vi "Know Position.vi"(0 "Ref_Drive 1R":T1, 1 "Ref_Drive 2R":T1, 2 "Ref_Drive 3R":T1, 3 "Ref_Drive 4L":T1, 4 "Ref_Drive 5L":T1, 5 "Ref_Drive 6L":T1) -> ()   [LabVIEW 2018]
uses:
  <vilib>/Rock Robotics/WPI/MotorControl/WPI_MotorControlDeviceRef.ctl
  <vilib>/Rock Robotics/WPI/MotorControl/WPI_MotorControlType.ctl
  <vilib>/Rock Robotics/SystemInterfaces/DIO/FPGA_DIOPWMChannel.ctl
  <vilib>/Rock Robotics/WPI/PWM/WPI_PWMDeadband.ctl
  <vilib>/Rock Robotics/SystemInterfaces/DIO/FPGA_DIOChannel.ctl
  Robot States.vi
  Sensor Readings.vi
panel:
  out "XY Graph":cluster{dbl[], dbl[]}(graph)
  in  "Reset Positon":bool
  out "Heading (deg)":dbl format="%#_13g"
  out "Y Position (in)":dbl
  out "X Position (in)":dbl
  in  "Plot Drive Encoder Data":bool
  out "Drive Encoder Velocities":cluster{dbl, dbl}
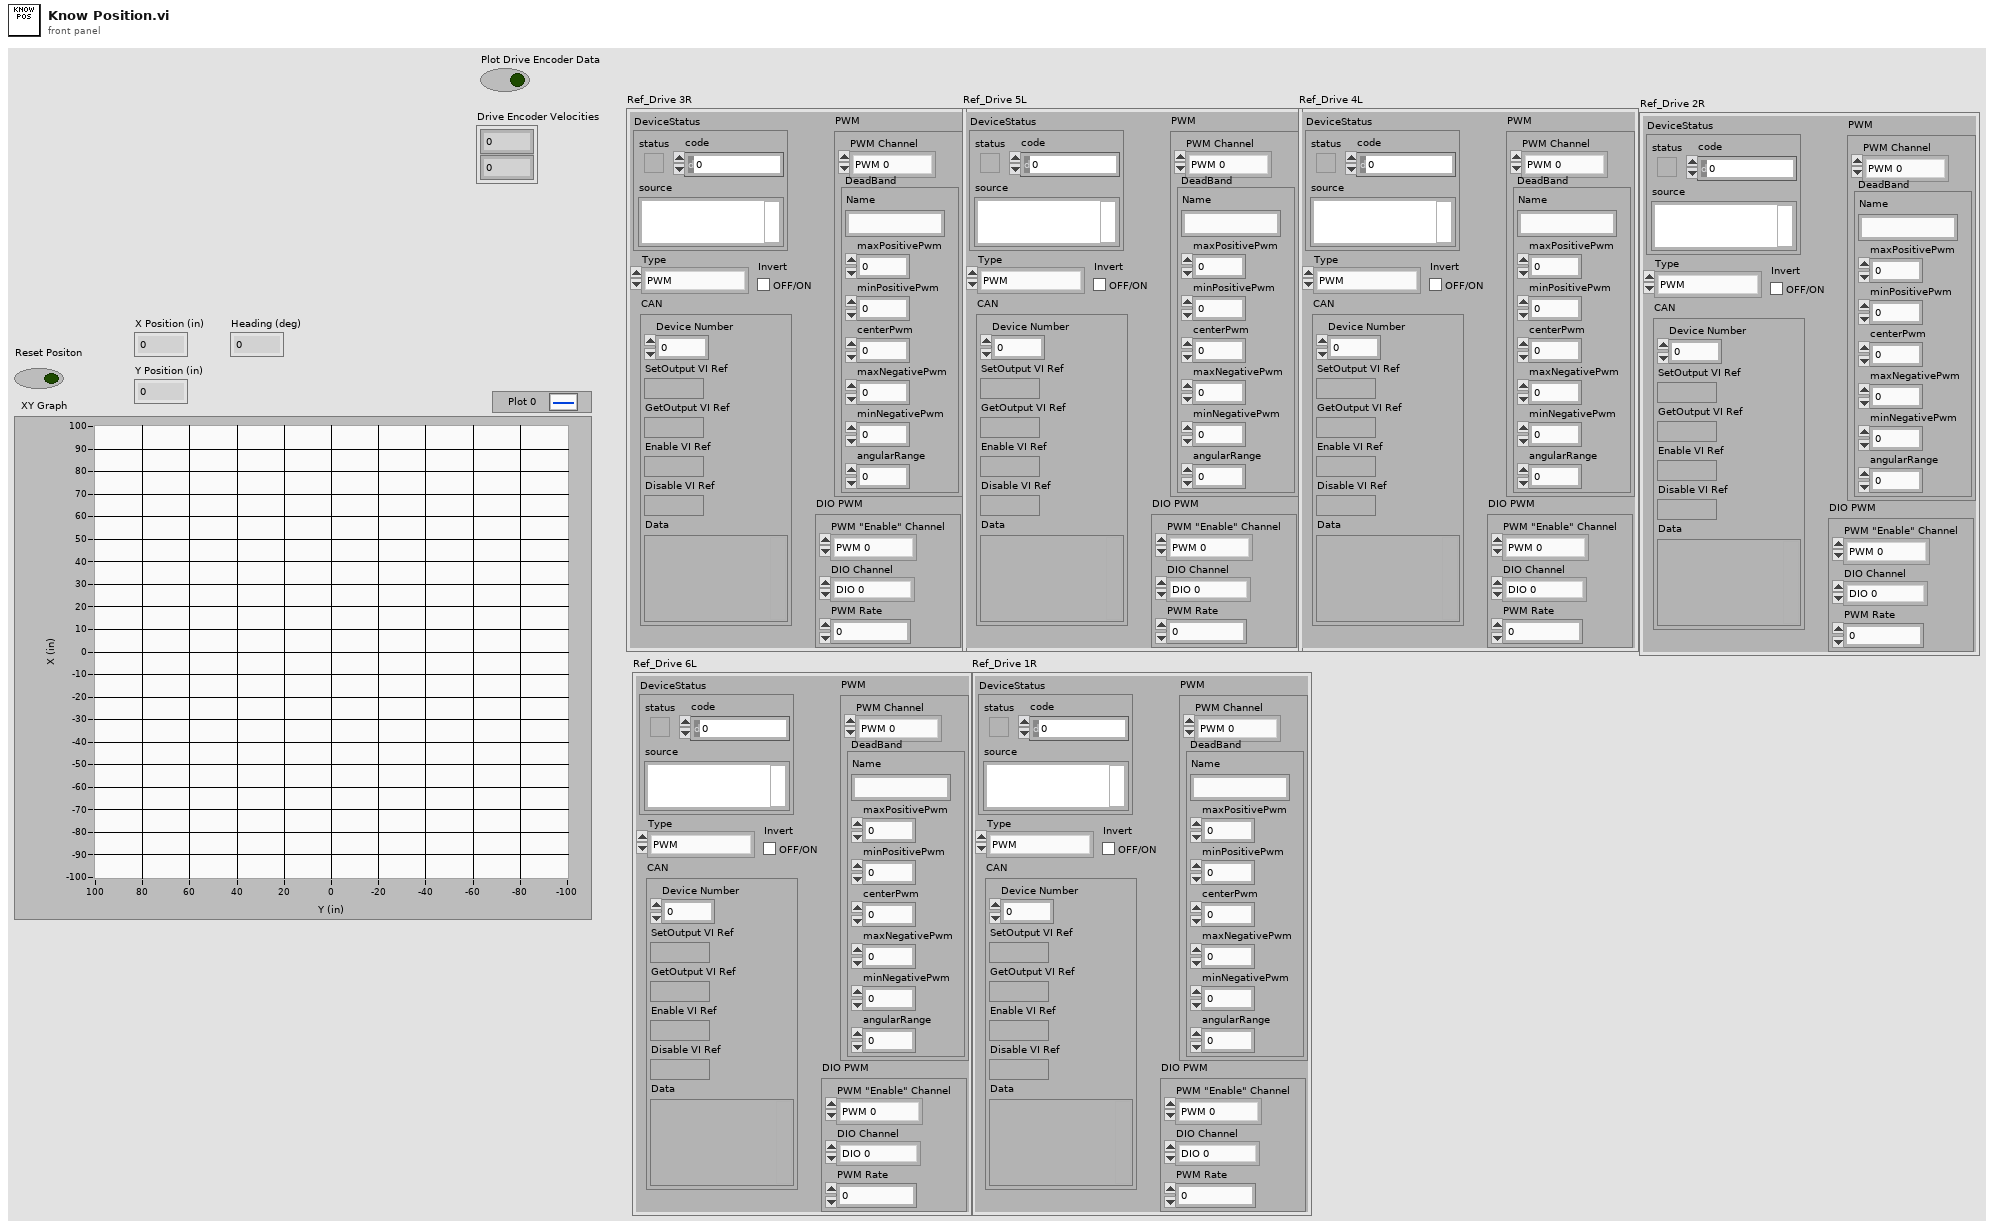
[diagram p1: front panel]
types:
  T1 = typedef "WPI_MotorControlDeviceRef.ctl" = cluster{"DeviceStatus":errorcluster, "Type":T2, "PWM":cluster{"PWM Channel":T3, "DeadBand":T4}, "CAN":cluster{"Device Number":u8, "SetOutput VI Ref":variant, "GetOutput VI Ref":variant, "Enable VI Ref":variant, "Disable VI Ref":variant, "Data":variant}, "Invert":bool, "DIO PWM":cluster{"PWM \"Enable\" Channel":T3, "DIOChannel":T5, "PWM Rate":dbl}}
  T2 = typedef "WPI_MotorControlType.ctl" = enum16{"PWM", "CAN", "DIO PWM"}
  T3 = typedef "FPGA_DIOPWMChannel.ctl" = enum8{"PWM 0", "PWM 1", "PWM 2", "PWM 3", "PWM 4", "PWM 5", "PWM 6", "PWM 7", "PWM 8", "PWM 9", "PWM MXP 0", "PWM MXP 1", "PWM MXP 2", "PWM MXP 3", "PWM MXP 4", "PWM MXP 5", "PWM MXP 6", "PWM MXP 7", "PWM MXP 8", "PWM MXP 9", "Invalid"}
  T4 = typedef "WPI_PWMDeadband.ctl" = cluster{"Name":string, "maxPositivePwm":i32, "minPositivePwm":i32, "centerPwm":i32, "maxNegativePwm":i32, "minNegativePwm":i32, "angularRange":u16}
  T5 = typedef "FPGA_DIOChannel.ctl" = enum8{"DIO 0", "DIO 1", "DIO 2", "DIO 3", "DIO 4", "DIO 5", "DIO 6", "DIO 7", "DIO 8", "DIO 9", "DIO MXP 0", "DIO MXP 1", "DIO MXP 2", "DIO MXP 3", "DIO MXP 4", "DIO MXP 5", "DIO MXP 6", "DIO MXP 7", "DIO MXP 8", "DIO MXP 9", "DIO MXP 10", "DIO MXP 11", "DIO MXP 12", "DIO MXP 13", "DIO MXP 14", "DIO MXP 15", "SPI Port CS1", "SPI Port CS2", "SPI Port CS3", "SPI Port MISO", "SPI Port MOSI", "Invalid"}
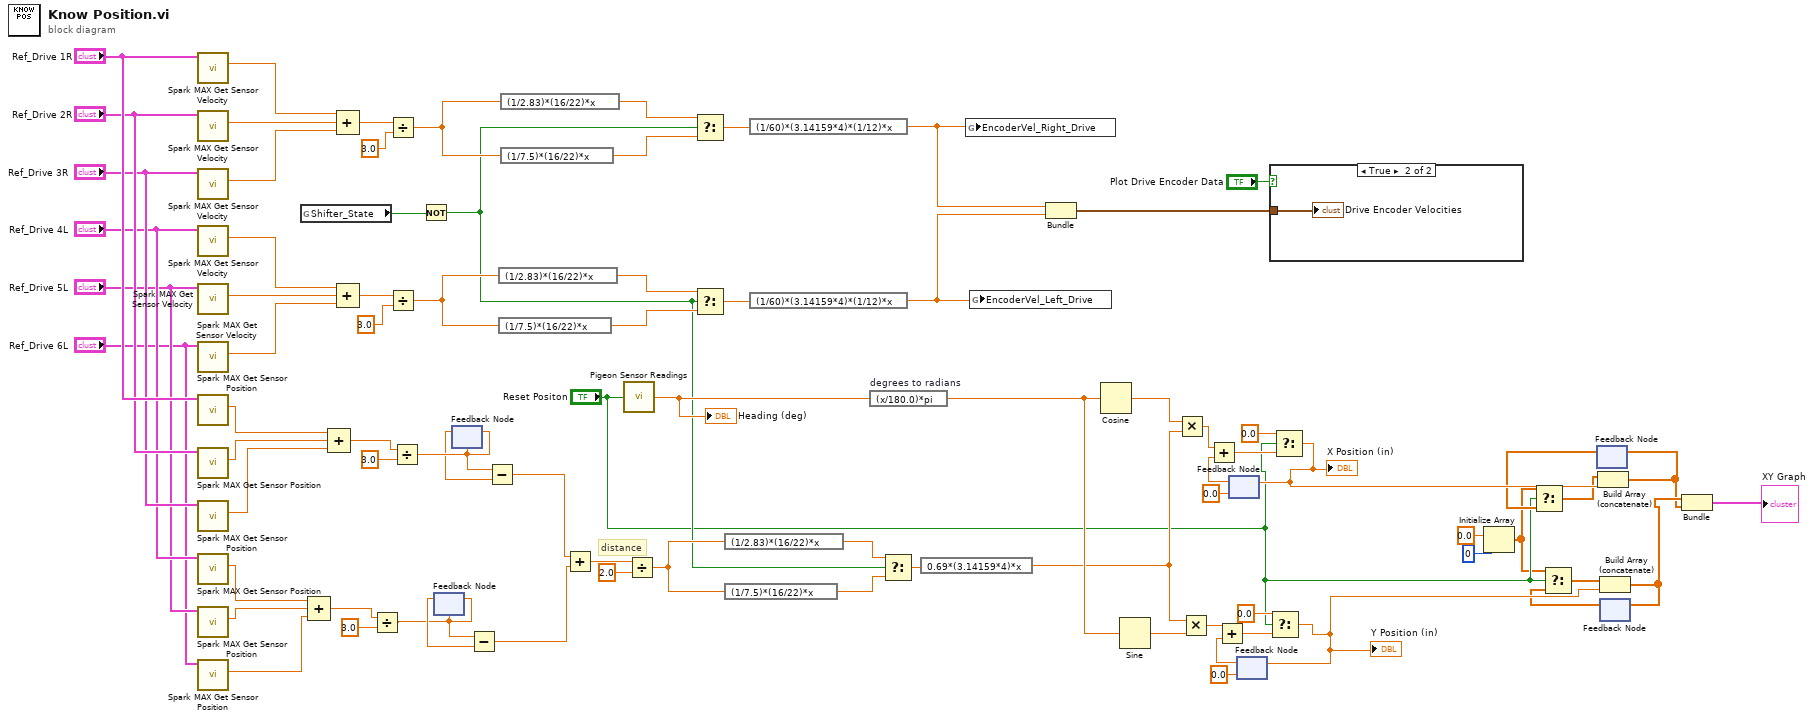
[diagram p0: block diagram]
diagram:
  # "distance"
  n1 = call <vilib>:"Spark MAX Get Sensor Velocity.vi"("MotorControlDevRef in"="Ref_Drive 1R") -> ("Sensor Velocity"=w80:dbl)  [unwired: 7 in, 3 out]
  n2 = call <vilib>:"Spark MAX Get Sensor Velocity.vi"("MotorControlDevRef in"="Ref_Drive 2R") -> ("Sensor Velocity"=w79:dbl)  [unwired: 7 in, 3 out]
  n3 = call <vilib>:"Spark MAX Get Sensor Velocity.vi"("MotorControlDevRef in"="Ref_Drive 3R") -> ("Sensor Velocity"=w78:dbl)  [unwired: 7 in, 3 out]
  n4 = call <vilib>:"Spark MAX Get Sensor Velocity.vi"("MotorControlDevRef in"="Ref_Drive 4L") -> ("Sensor Velocity"=w77:dbl)  [unwired: 7 in, 3 out]
  n5 = call <vilib>:"Spark MAX Get Sensor Velocity.vi"("MotorControlDevRef in"="Ref_Drive 5L") -> ("Sensor Velocity"=w76:dbl)  [unwired: 7 in, 3 out]
  n6 = call <vilib>:"Spark MAX Get Sensor Velocity.vi"("MotorControlDevRef in"="Ref_Drive 6L") -> ("Sensor Velocity"=w75:dbl)  [unwired: 7 in, 3 out]
  n7 = call <vilib>:"Spark MAX Get Sensor Position.vi"("MotorControlDevRef in"="Ref_Drive 1R") -> ("Sensor Position"=w51:dbl)  [unwired: 7 in, 3 out]
  n8 = call <vilib>:"Spark MAX Get Sensor Position.vi"("MotorControlDevRef in"="Ref_Drive 2R") -> ("Sensor Position"=w50:dbl)  [unwired: 7 in, 3 out]
  n9 = call <vilib>:"Spark MAX Get Sensor Position.vi"("MotorControlDevRef in"="Ref_Drive 3R") -> ("Sensor Position"=w49:dbl)  [unwired: 7 in, 3 out]
  n10 = call <vilib>:"Spark MAX Get Sensor Position.vi"("MotorControlDevRef in"="Ref_Drive 4L") -> ("Sensor Position"=w44:dbl)  [unwired: 7 in, 3 out]
  n11 = call <vilib>:"Spark MAX Get Sensor Position.vi"("MotorControlDevRef in"="Ref_Drive 5L") -> ("Sensor Position"=w43:dbl)  [unwired: 7 in, 3 out]
  n12 = call <vilib>:"Spark MAX Get Sensor Position.vi"("MotorControlDevRef in"="Ref_Drive 6L") -> ("Sensor Position"=w42:dbl)  [unwired: 7 in, 3 out]
  n13 = global read "Robot States.vi" "Shifter_State"() -> (w70:bool)
  n14 = Compound Arithmetic op=ADD(w44, w43, w42) -> (w46:dbl)
  n15 = Compound Arithmetic op=ADD(w51, w50, w49) -> (w48:dbl)
  n16 = Compound Arithmetic op=ADD(w80, w79, w78) -> (w72:dbl)
  n17 = Compound Arithmetic op=ADD(w77, w76, w75) -> (w71:dbl)
  n18 = Divide(x=w46, y=3.0) -> (x/y=w21:dbl)
  n19 = Divide(x=w72, y=3.0) -> (x/y=w68:dbl)
  n20 = Divide(x=w71, y=3.0) -> (x/y=w69:dbl)
  n21 = Divide(x=w48, y=3.0) -> (x/y=w25:dbl)
  n22 = Not(x=w70) -> (.not. x?=w26:bool)
  n23 = feedback #1(w21) -> (w22:dbl)
  n24 = feedback-in #1(w21) -> ()
  n25 = feedback-in #2(w25) -> ()
  n26 = feedback #2(w25) -> (w24:dbl)
  n27 = Subtract(x=w21, y=w22) -> (x-y=w20:dbl)
  n28 = Subtract(x=w25, y=w24) -> (x-y=w23:dbl)
  n29 = expression code="(1/2.83)*(16/22)*x"(w69) -> (w65:dbl)
  n30 = expression code="(1/7.5)*(16/22)*x"(w69) -> (w64:dbl)
  n31 = expression code="(1/2.83)*(16/22)*x"(w68) -> (w67:dbl)
  n32 = expression code="(1/7.5)*(16/22)*x"(w68) -> (w66:dbl)
  n33 = Add(x=w23, y=w20) -> (x+y=w41:dbl)
  n34 = call "Pigeon Sensor Readings.vi"("Reset Yaw"="Reset Positon") -> ("Yaw"=w31:dbl)
  "Heading (deg)" <- w31
  n35 = Divide(x=w41, y=2.0) -> (x/y=w27:dbl)
  n36 = Select(t=w67, s=w26, f=w66) -> (s? t:f=w63:dbl)
  n37 = Select(t=w65, s=w26, f=w64) -> (s? t:f=w62:dbl)
  n38 = expression code="(1/2.83)*(16/22)*x"(w27) -> (w29:dbl)
  n39 = expression code="(1/7.5)*(16/22)*x"(w27) -> (w28:dbl)
  n40 = expression code="(1/60)*(3.14159*4)*(1/12)*x"(w63) -> (w61:dbl)
  n41 = expression code="(1/60)*(3.14159*4)*(1/12)*x"(w62) -> (w60:dbl)
  n42 = expression code="(x/180.0)*pi" "degrees to radians"(w31) -> (w30:dbl)
  n43 = Select(t=w29, s=w26, f=w28) -> (s? t:f=w15:dbl)
  n44 = expression code="0.69*(3.14159*4)*x"(w15) -> (w14:dbl)
  n45 = global write "Sensor Readings.vi" "EncoderVel_Right_Drive"(w61) -> ()
  n46 = global write "Sensor Readings.vi" "EncoderVel_Left_Drive"(w60) -> ()
  n47 = Bundle(w61, w60) -> (w58:cluster{dbl, dbl})  [unwired: 1 in]
  n48 = Cosine(x=w30) -> (cos(x)=w39:dbl)
  n49 = Sine(x=w30) -> (sin(x)=w38:dbl)
  n50 = Multiply(x=w39, y=w14) -> (x*y=w37:dbl)
  n51 = Multiply(x=w14, y=w38) -> (x*y=w35:dbl)
  n52 = feedback #3(0.0) -> (w36:dbl)
  n53 = Add(x=w37, y=w36) -> (x+y=w17:dbl)
  n54 = feedback #4(0.0) -> (w34:dbl)
  n55 = Add(x=w35, y=w34) -> (x+y=w19:dbl)
  n56 = case shown="True" "Plot Drive Encoder Data" {
    tunnel: w58 -> [_ w81]
    frame False {
    }
    frame True {
      "Drive Encoder Velocities" <- w81
    }
  }
  n57 = Select(t=0.0, s="Reset Positon", f=w19) -> (s? t:f=w12:dbl)
  "Y Position (in)" <- w12
  n58 = feedback-in #4(w12) -> ()
  n59 = Select(t=0.0, s="Reset Positon", f=w17) -> (s? t:f=w11:dbl)
  "X Position (in)" <- w11
  n60 = feedback-in #3(w11) -> ()
  n61 = Initialize Array(0.0 ("element"), 0 ("dimension size")) -> (w1:dbl[])
  n62 = feedback #5() -> (w8:dbl[])  [unwired: 1 in]
  n63 = Select(t=w1, s="Reset Positon", f=w8) -> (s? t:f=w7:dbl[])
  n64 = Build Array (concatenate)(w7, w11) -> (w9:dbl[])
  n65 = feedback-in #5(w9) -> ()
  n66 = feedback #6() -> (w6:dbl[])  [unwired: 1 in]
  n67 = Select(t=w1, s="Reset Positon", f=w6) -> (s? t:f=w5:dbl[])
  n68 = Build Array (concatenate)(w5, w12) -> (w10:dbl[])
  n69 = feedback-in #6(w10) -> ()
  n70 = Bundle(w10, w9) -> (→"XY Graph":cluster{dbl[], dbl[]})  [unwired: 1 in]
